vi "get path to audit barcode formats.vi"(10 "product":string, 11 "paths.Base Path":path) -> (3 "path":path)   [LabVIEW 2018]
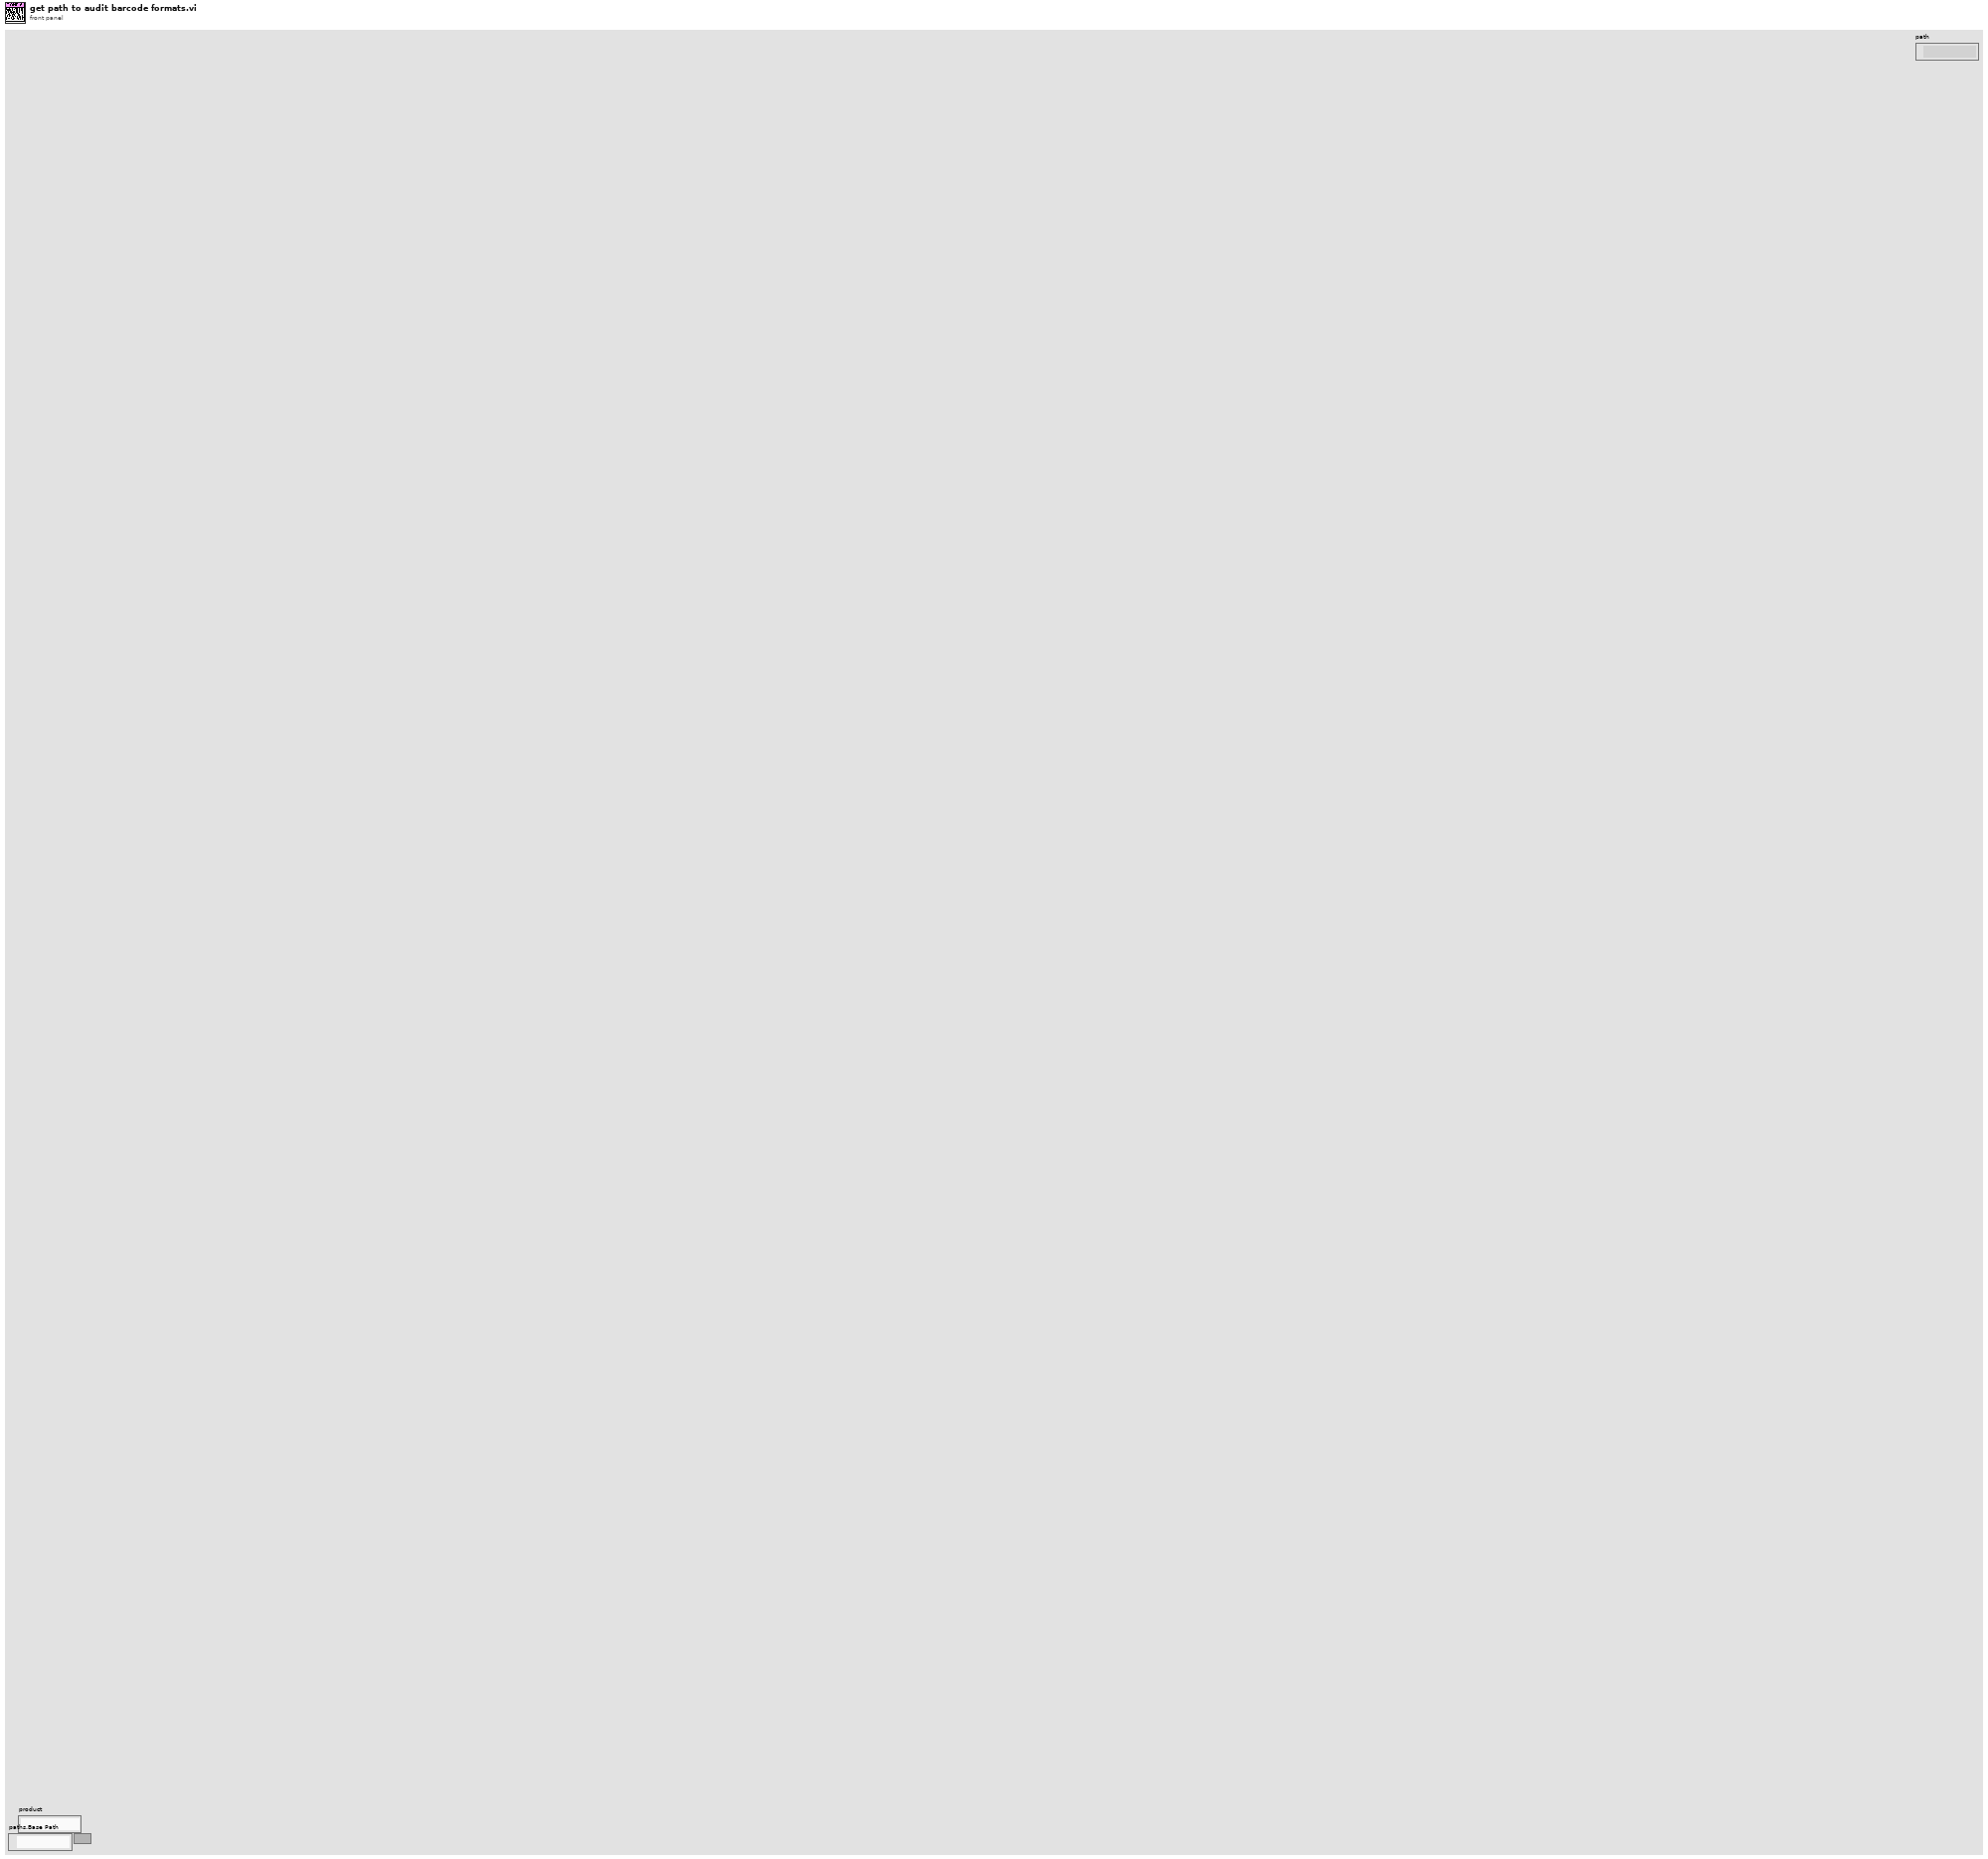
[diagram p1: front panel]
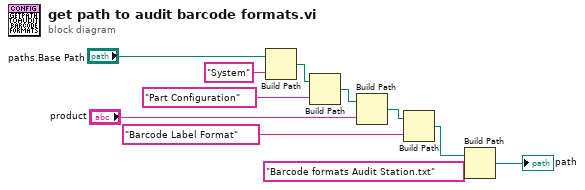
[diagram p0: block diagram]
diagram:
  n1 = Build Path(base path="paths.Base Path", name or relative path="System") -> (appended path=w7:path)
  n2 = Build Path(base path=w7, name or relative path="Part Configuration") -> (appended path=w8:path)
  n3 = Build Path(base path=w8, name or relative path="product") -> (appended path=w9:path)
  n4 = Build Path(base path=w9, name or relative path="Barcode Label Format") -> (appended path=w3:path)
  n5 = Build Path(base path=w3, name or relative path="Barcode formats Audit Station.txt") -> (appended path=→"path":path)
